vi "Save_Automation_Test.vi"(7 "Resultados":T1, 11 "error in (no error)":errorcluster) -> (15 "error out":errorcluster)   [LabVIEW 2021]
uses:
  Type defs/Table_Result_Automation_Test.ctl
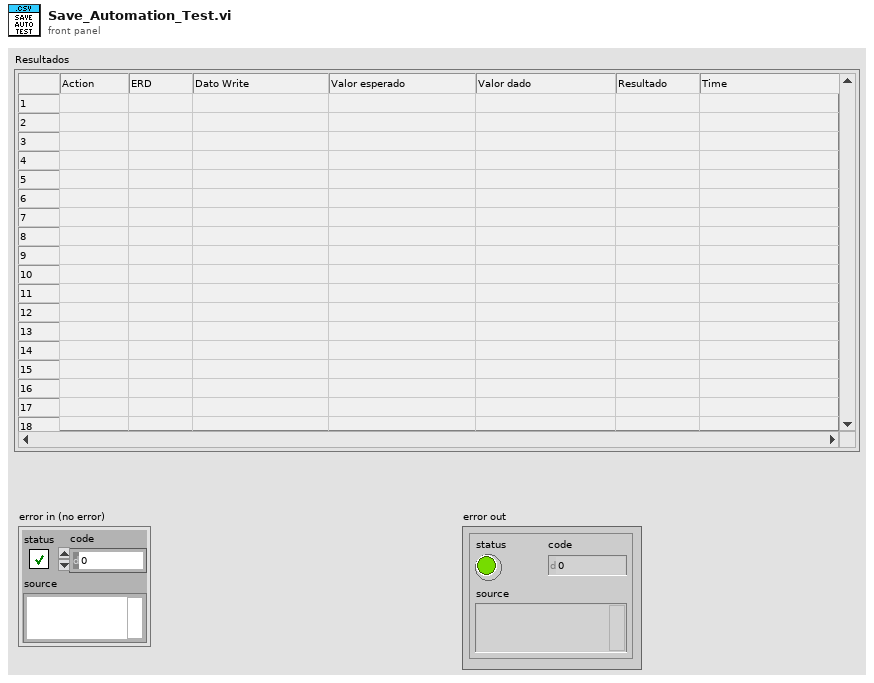
[diagram p1: front panel]
types:
  T1 = typedef "Table_Result_Automation_Test.ctl" = string[][]
  T2 = enum16{"open", "replace", "create", "open or create", "replace or create", "replace or create with confirmation"}
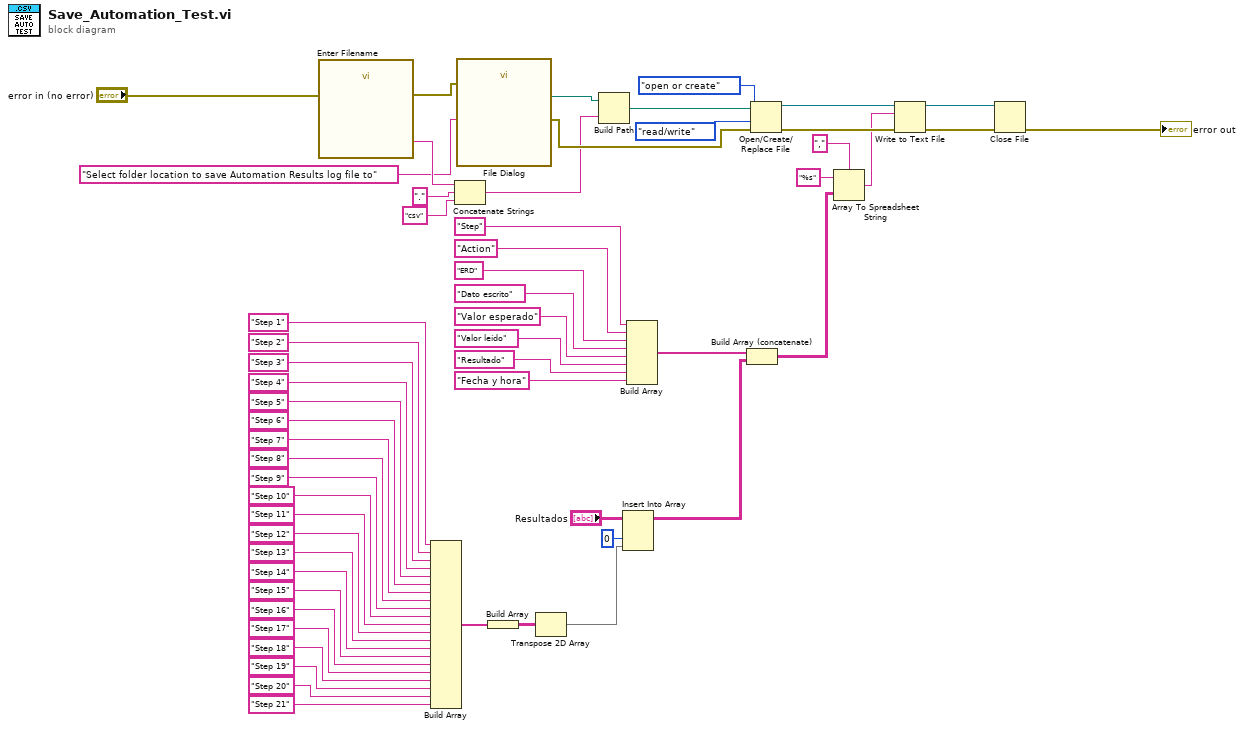
[diagram p0: block diagram]
diagram:
  n1 = call "Enter Filename"("error in (no error)"="error in (no error)") -> ("Filename"=w55:string, "error out"=w50:errorcluster)  [unwired: 16 in, 1 out]
  n2 = Build Array("Step 1", "Step 2", "Step 3", "Step 4", "Step 5", "Step 6", "Step 7", "Step 8", "Step 9", "Step 10", "Step 11", "Step 12", "Step 13", "Step 14", "Step 15", "Step 16", "Step 17", "Step 18", "Step 19", "Step 20", "Step 21") -> (w28:string[])
  n3 = Concatenate Strings(w55, "." ("string"), "csv" ("string")) -> (w54:string)
  n4 = call "File Dialog"("prompt"="Select folder location to save Automation Results log file to", "error in"=w50) -> ("selected path"=w47:path, "error out"=w56:errorcluster)  [unwired: 10 in, 2 out]
  n5 = Build Array(w28) -> (w27:string[][])
  n6 = Transpose 2D Array(2D array=w27) -> (transposed array=w25:string[][])
  n7 = Build Path(base path=w47, name or relative path=w54) -> (appended path=w48:path)
  n8 = Insert Into Array(array="Resultados", index (col)=0 ("disabled index (col)"), new element=w25) -> (w4:T1)  [unwired: 1 in]
  n9 = Build Array("Step", "Action" ("element"), "ERD" ("element"), "Dato escrito" ("element"), "Valor esperado" ("element"), "Valor leído" ("element"), "Resultado" ("element"), "Fecha y hora" ("element")) -> (w30:string[])
  n10 = Build Array (concatenate)(w30, w4) -> (w2:T1)
  n11 = Open/Create/Replace File(file path (use dialog)=w48, error in=w56, operation (0:open)=T2."open or create", access (0:read/write)=enum16{"read/write", "read-only", "write-only"}."read/write") -> (refnum out=w46:refnum<file>, error out=w45:errorcluster)  [unwired: 2 in, 1 out]
  n12 = Array To Spreadsheet String(delimiter (Tab)=",", array=w2, 3:"%s" ("format string")) -> (spreadsheet string=w41:string)
  n13 = Write to Text File(file (use dialog)=w46, text=w41, error in=w45) -> (refnum out=w44:refnum<file>, error out=w43:errorcluster)  [unwired: 1 in, 1 out]
  n14 = Close File(refnum=w44, error in=w43) -> (error out=→"error out":errorcluster)  [unwired: 1 out]
